vi "Build Tree.vi"(8 "error in (no error)":errorcluster, 9 "Wired-in Class Refnum":refnum<vi>, 10 "Method Name":string, 11 "Tree Refnum":refnum<vi>) -> (0 "error out":errorcluster, 2 "All Classes":refnum<vi>[](array[refnum]), 3 "Tree Refnum out":refnum<vi>)   [LabVIEW 2020, in "Choose Implementation Dialog.lvlib"]
uses:
  Choose Implementation Dialog.lvlib
  Tree Item Info.ctl
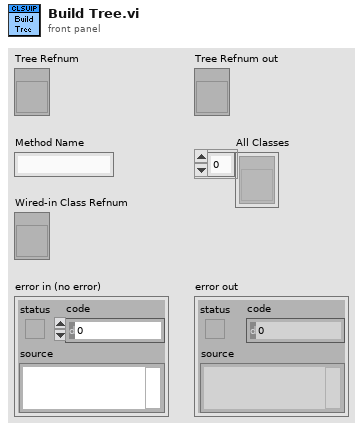
[diagram p1: front panel]
types:
  T1 = typedef "Choose Implementation Dialog.lvlib/Tree Item Info.ctl" = cluster{"ClassRef":refnum<vi>, "Implementor?":bool, "Parent ItemID":string}
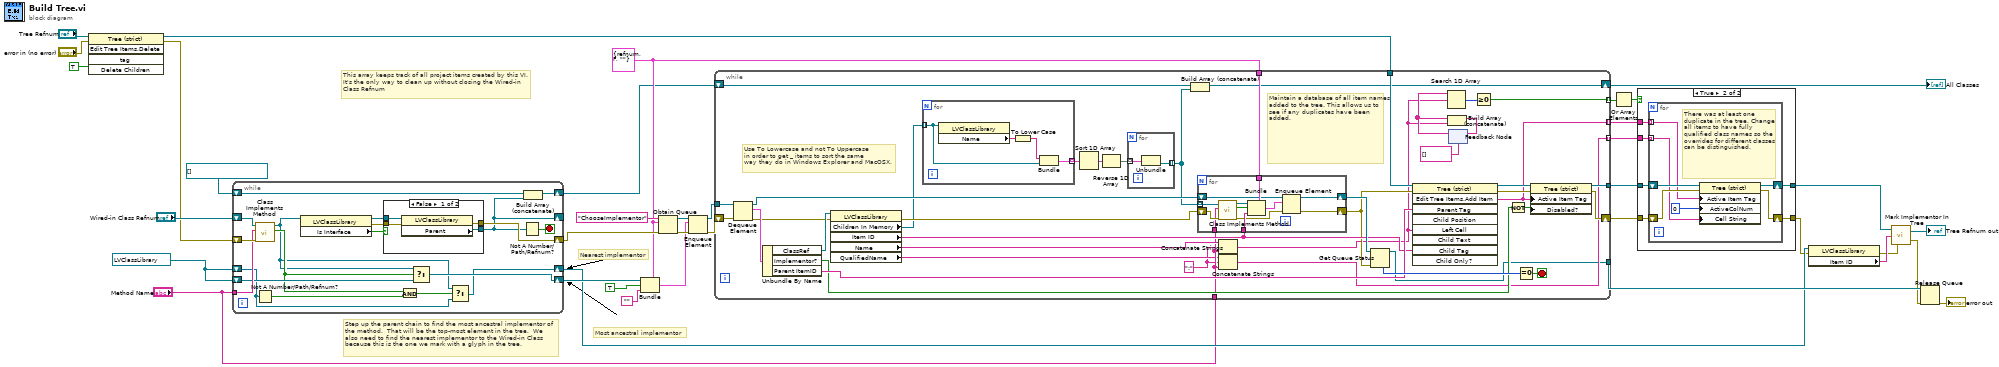
[diagram p0: block diagram]
diagram:
  w16 = refnum<vi> refnum ("Class Refnum out")
  w27 = T1 {"ClassRef"=refnum, "Implementor?"=FALSE, "Parent ItemID"=""} ("Cluster")
  # "This array keeps track of all project items created by this VI.\nIt's the only way to clean up without closing the Wired-in \nClass Refnum"
  # "Most ancestral implementor"
  # "Nearest implementor"
  # "Step up the parent chain to find the most ancestral implementor of\nthe method.  That will be the top-most element in the tree.  We\nalso need to find the nearest implementor to the Wired-in Class\nbecause this is the one we mark with a glyph in the tree."
  n1 = invoke class="Tree (strict)" method="Edit Tree Items.Delete"(reference="Tree Refnum", error in="error in (no error)", "Delete Children"=TRUE ("Delete Children?")) -> (reference out=w25:refnum<vi>, error out=w1:errorcluster)  [unwired: 2 in, 3 out]
  n2 = while {
    shift-right: [w51] -> w37
    shift-left: w16 -> [w52]
    shift-right: [w44] -> _
    shift-left: "Wired-in Class Refnum" -> [w54]
    shift-right: [w45] -> w35
    shift-left: w1 -> [w55]
    tunnel: "Method Name" -> [w53]
    shift-right: [w46] -> w18
    shift-left: w16 -> [w47]
    shift-right: [w42] -> w13
    shift-left: refnum<vi>[] [] -> [w43]
    stop <- w56 stop-if-true
    n3 = call "Class Implements Method.vi"("error in (no error)"=w55, "Method Name"=w53, "Class Refnum"=w54) -> ("Implements method?"=w49:bool, "Class Refnum out"=w39:refnum<vi>)  [unwired: 6 in, 1 out]
    n4 = Not A Number/Path/Refnum?(number/path/refnum=w47) -> (NaN/Path/Refnum?=w50:bool)
    n5 = property class="LVClassLibrary"(reference=w39) -> (reference out=w41:refnum<vi>, error out=w40:errorcluster, "Is Interface"=w38:bool)  [unwired: 1 in]
    n6 = case shown="False" w38 {
      tunnel: [w60 w61] -> w45
      tunnel: [w59 _] -> w44
      tunnel: w41 -> [w58 _]
      tunnel: w40 -> [w57 w61]
      frame False {
        n7 = property class="LVClassLibrary"(reference=w58, error in=w57) -> (error out=w60:errorcluster, "Parent"=w59:refnum<vi>)  [unwired: 1 out]
      }
      frame True {
      }
    }
    n8 = And(x=w49, y=w50) -> (x .and. y?=w48:bool)
    n9 = Select(t=w39, s=w49, f=w52) -> (s? t:f=w51:refnum<vi>)
    n10 = Select(t=w39, s=w48, f=w47) -> (s? t:f=w46:refnum<vi>)
    n11 = Not A Number/Path/Refnum?(number/path/refnum=w44) -> (NaN/Path/Refnum?=w56:bool)
    n12 = Build Array (concatenate)(w43, w44) -> (w42:refnum<vi>[])
  }
  n13 = Bundle(cluster=w27, "ClassRef"=w37, "Implementor?"=TRUE, "Parent ItemID"="") -> (w31:T1)
  n14 = Obtain Queue(name (unnamed)="ChooseImplementor", element data type=w27, error in (no error)=w35) -> (queue out=w33:refnum<queue>, error out=w32:errorcluster)  [unwired: 2 in, 1 out]
  n15 = Enqueue Element(queue=w33, element=w31, error in (no error)=w32) -> (queue out=w30:refnum<queue>, error out=w29:errorcluster)  [unwired: 1 in, 1 out]
  n16 = while {
    tunnel: w30 -> [w102]
    shift-right: [w83] -> w6
    shift-left: w29 -> [w101]
    tunnel: w27 -> [w93]
    tunnel: "Method Name" -> [w72]
    tunnel: w25 -> [w91]
    tunnel: [w82] -> w8
    tunnel: [w62] -> w21
    shift-right: [w79] -> w11
    shift-left: w13 -> [w80]
    tunnel: [w73] -> w4 mode=indexing
    tunnel: [w67] -> w3 mode=indexing
    tunnel: [w63] -> w10 mode=indexing
    stop <- w100 stop-if-true
    w70 = ":" ("element")
    # "Maintain a database of all item names added to the tree. This allows us to see if any duplicates have been added."
    # "Use To Lowercase and not To Uppercase\nin order to get _ items to sort the same\nway they do in Windows Explorer and MacOSX."
    n17 = Dequeue Element(queue=w102, error in (no error)=w101) -> (queue out=w95:refnum<queue>, element=w98:T1, error out=w96:errorcluster)  [unwired: 1 in, 1 out]
    n18 = Unbundle By Name(w98) -> ("ClassRef"=w97:refnum<vi>, "Implementor?"=w84:bool, "Parent ItemID"=w89:string)
    n19 = property class="LVClassLibrary"(reference=w97, error in=w96) -> (error out=w94:errorcluster, "Children In Memory"=w76:refnum<vi>[], "Item ID"=w88:string, "Name"=w90:string, "QualifiedName"=w71:string)  [unwired: 1 out]
    n20 = for {
      tunnel: w76 -> [w107] mode=indexing
      tunnel: [w106] -> w78 mode=indexing
      n21 = property class="LVClassLibrary"(reference=w107) -> ("Name"=w108:string)  [unwired: 1 in, 2 out]
      n22 = To Lower Case(string=w108) -> (all lower case string=w105:string)
      n23 = Bundle(w105, w107) -> (w106:cluster{string, refnum<vi>})  [unwired: 1 in]
    }
    n24 = Sort 1D Array(array=w78) -> (sorted array=w77:cluster{string, refnum<vi>}[])
    n25 = Reverse 1D Array(array=w77) -> (reversed array=w74:cluster{string, refnum<vi>}[])
    n26 = for {
      tunnel: w74 -> [w104] mode=indexing
      tunnel: [w103] -> w75 mode=indexing
      n27 = Unbundle(w104) -> (w103:refnum<vi>)  [unwired: 1 out]
    }
    n28 = Build Array (concatenate)(w80, w75) -> (w79:refnum<vi>[])
    n29 = for {
      tunnel: w75 -> [w115] mode=indexing
      shift-right: [w109] -> w81
      shift-left: w94 -> [w114]
      tunnel: w93 -> [w120]
      tunnel: w88 -> [w117]
      tunnel: w72 -> [w113]
      shift-right: [w112] -> w92
      shift-left: w95 -> [w119]
      n30 = call "Class Implements Method.vi"("error in (no error)"=w114, "Method Name"=w113, "Class Refnum"=w115) -> ("error out"=w111:errorcluster, "Implements method?"=w116:bool, "Class Refnum out"=w110:refnum<vi>)  [unwired: 6 in]
      n31 = Bundle(cluster=w120, "ClassRef"=w110, "Implementor?"=w116, "Parent ItemID"=w117) -> (w118:T1)
      n32 = Enqueue Element(queue=w119, element=w118, error in (no error)=w111) -> (queue out=w112:refnum<queue>, error out=w109:errorcluster)  [unwired: 1 in, 1 out]
    }
    n33 = Concatenate Strings(w90, w70, w72) -> (w65:string)
    n34 = Concatenate Strings(w71, w70, w72) -> (w67:string)
    n35 = Get Queue Status(queue=w92, error in (no error)=w81) -> (queue out=w62:refnum<queue>, # elements in queue=w99:i32)  [unwired: 1 in, 6 out]
    n36 = invoke class="Tree (strict)" method="Edit Tree Items.Add Item"(reference=w91, error in=w81, "Parent Tag"=w89, "Left Cell"=w65, "Child Tag"=w88) -> (reference out=w87:refnum<vi>, error out=w86:errorcluster, "Edit Tree Items:Add Item"=w73:string)  [unwired: 4 in, 6 out]
    n37 = feedback #1(string[] []) -> (w66:string[])
    n38 = Search 1D Array(1D array=w66, element=w65) -> (index of element=w64:i32)  [unwired: 1 in]
    n39 = Build Array (concatenate)(w66, w65) -> (w68:string[])
    n40 = feedback-in #1(w68) -> ()
    n41 = Greater Or Equal To 0?(x=w64) -> (x >= 0?=w63:bool)
    n42 = Not(x=w84) -> (.not. x?=w85:bool)
    n43 = Equal To 0?(x=w99) -> (x = 0?=w100:bool)
    n44 = property class="Tree (strict)"(reference=w87, error in=w86, "Active Item Tag"=w73, "Disabled?"=w85) -> (reference out=w82:refnum<vi>, error out=w83:errorcluster)
  }
  "All Classes" <- w11
  n45 = Or Array Elements(Boolean array=w10) -> (logical OR=w9:bool)
  n46 = case shown="True" w9 {
    tunnel: w8 -> [w122 w126]
    tunnel: [w122 w125] -> w7
    tunnel: w6 -> [w121 w124]
    tunnel: [w121 w123] -> w5
    tunnel: w4 -> [_ w128]
    tunnel: w3 -> [_ w127]
    frame False {
      # "No duplicate items in the tree, no need to update class file names in the tree to qualified class names."
    }
    frame True {
      n47 = for {
        tunnel: w128 -> [w131] mode=indexing
        tunnel: w127 -> [w129] mode=indexing
        shift-right: [w134] -> w125
        shift-left: w126 -> [w135]
        shift-right: [w132] -> w123
        shift-left: w124 -> [w133]
        # "There was at least one duplicate in the tree. Change all items to have fully qualified class names so the overrides for different classes can be distinguished."
        n48 = property class="Tree (strict)"(reference=w135, error in=w133, "Active Item Tag"=w131, "ActiveColNum"=0 ("Active Cell:Active Column Number"), "Cell String"=w129) -> (reference out=w134:refnum<vi>, error out=w132:errorcluster)
      }
    }
  }
  n49 = property class="LVClassLibrary"(reference=w18, error in=w5) -> (error out=w12:errorcluster, "Item ID"=w17:string)  [unwired: 1 out]
  n50 = call "Mark Implementor In Tree.vi"("error in (no error)"=w12, "Item ID to mark"=w17, "Tree Refnum in"=w7) -> ("error out"=w20:errorcluster, "Tree Refnum out"=→"Tree Refnum out":refnum<vi>)
  n51 = Release Queue(queue=w21, error in (no error)=w20) -> (error out=→"error out":errorcluster)  [unwired: 1 in, 2 out]
